vi "bytes_to_bits.vi"(2 "Numeric":i8) -> (1 "bit 1":bool, 4 "bit 8":bool, 5 "bit 2":bool, 6 "bit 3":bool, 7 "bit 4":bool, 8 "bit 7":bool, 9 "bit 5":bool, 10 "bit 6":bool)   [LabVIEW 2010]
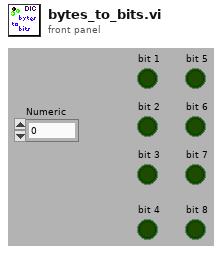
[diagram p1: front panel]
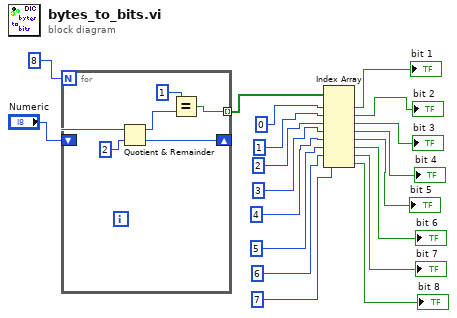
[diagram p0: block diagram]
diagram:
  n1 = for {
    N: 8 -> [_]
    shift-right: [w24] -> _
    shift-left: "Numeric" -> [w25]
    tunnel: [w21] -> w17 mode=indexing
    n2 = Quotient & Remainder(x=w25, y=2) -> (x-y*floor(x/y)=w22:i32, floor(x/y)=w24:i32)
    n3 = Equal?(x=1, y=w22) -> (x = y?=w21:bool)
  }
  n4 = Index Array(array=w17, index #1=0, index #2=1, index #3=2, index #4=3, index #5=4, index #6=5, index #7=6, index #8=7) -> (element #1=→"bit 1":bool, element #2=→"bit 2":bool, element #3=→"bit 3":bool, element #4=→"bit 4":bool, element #5=→"bit 5":bool, element #6=→"bit 6":bool, element #7=→"bit 7":bool, element #8=→"bit 8":bool)
